vi "get call chain.vi"(11 "exception in":T1 {"code" format="%.0x"}) -> (2 "call chain":string[](array[string]), 3 "exception out":T1 {"code" format="%.0x"})   [LabVIEW 2013, in "exception.lvlib"]
uses:
  exception.lvlib
  exception.ctl
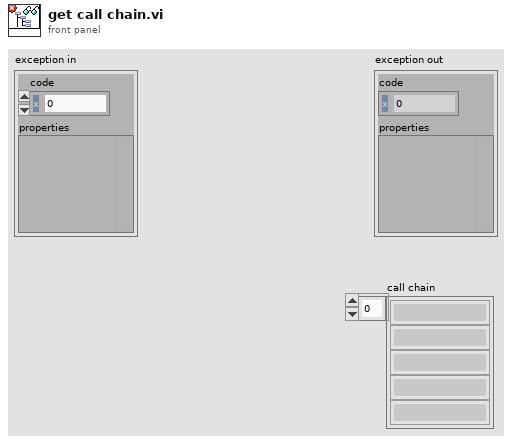
[diagram p1: front panel]
types:
  T1 = typedef "exception.lvlib/exception.ctl" = cluster{"code":i32, "properties":variant}
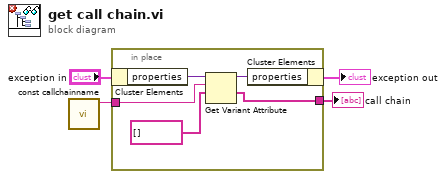
[diagram p0: block diagram]
diagram:
  n1 = call "const callchainname.vi"() -> ("label"=w2:string)  [unwired: 11 in]
  n2 = in-place {
    in-place-border: w2 -> [w7]
    in-place-border: [w5] -> w1
    n3 = in-place-cluster #1("exception in") -> ("properties"=w9:variant)
    n4 = Get Variant Attribute(Variant=w9, name=w7, default value (empty Variant)=string[] [] ("call chain")) -> (duplicate Variant=w8:variant, value=w5:string[])  [unwired: 1 in, 2 out]
    n5 = in-place-cluster #1("properties"=w8) -> (→"exception out":T1)
  }
  "call chain" <- w1
